vi "Find Entity by ID.vi"(7 "Entity Type":refnum<class "Entity.lvclass">, 8 "error in (no error)":errorcluster, 10 "Entity ID":T1, 11 "Entity Manager in":refnum<class "Entity Manager.lvclass">) -> (0 "error out":errorcluster, 2 "Entity":refnum<class "Entity.lvclass">, 3 "Entity Manager out":refnum<class "Entity Manager.lvclass">)   [LabVIEW 2020, in "Conditu2.lvlib" / "Entity Manager.lvclass"]
uses:
  Entity Manager.lvclass
  Entity/Entity.lvclass
  Entity ID.ctl
  Entity Manager.lvclass/Entity Manager.ctl
  Unit Of Work Session/Unit Of Work Session.lvclass
  Conditu2.lvlib
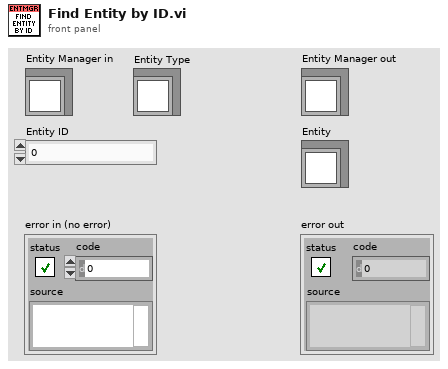
[diagram p1: front panel]
types:
  T1 = typedef "Conditu2.lvlib/Entity ID.ctl" = i64
  T2 = typedef "Conditu2.lvlib/Entity Manager.lvclass/Entity Info.ctl" = cluster{"Entity":refnum<class "Entity.lvclass">, "Types":refnum<class "Type.lvclass">[], "Type Name Map":map{string, i32}, "Has Relation":bool}
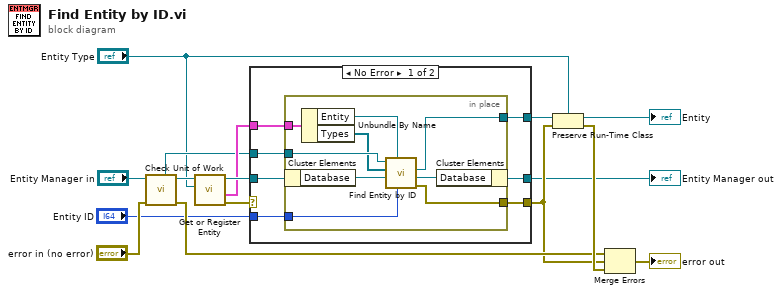
[diagram p0: block diagram]
diagram:
  n1 = call "Check Unit of Work.vi"("error in (no error)"="error in (no error)", "Entity Manager in"="Entity Manager in") -> ("error out"=w15:errorcluster, "Entity Manager out"=w4:refnum<class "Entity Manager.lvclass">, "Unit Of Work"=w3:refnum<class "Unit Of Work Session.lvclass">)  [unwired: 7 in]
  n2 = call "Get or Register Entity.vi"("Entity"="Entity Type", "Entity Manager in"=w4) -> ("error out"=w7:errorcluster, "Entity Info"=w9:T2, "Entity Manager out"=w10:refnum<class "Entity Manager.lvclass">)  [unwired: 7 in]
  n3 = case shown="No Error" w7 {
    selector: w7 -> [_ w34]
    tunnel: [w17 w34] -> w13
    tunnel: "Entity ID" -> [w23 _]
    tunnel: [w22 w33] -> w11
    tunnel: w10 -> [w20 w33]
    tunnel: w9 -> [w21 _]
    tunnel: w3 -> [w19 _]
    tunnel: [w18 _] -> w1
    frame No Error {
      n4 = in-place {
        in-place-border: w23 -> [w29]
        in-place-border: w21 -> [w32]
        in-place-border: w19 -> [w30]
        in-place-border: [w27] -> w18
        in-place-border: [w28] -> w17
        n5 = in-place-cluster #1(w20) -> ("Database"=w24:refnum<class "Database Platform.lvclass">)
        n6 = Unbundle By Name(w32) -> ("Entity"=w31:refnum<class "Entity.lvclass">, "Types"=w25:refnum<class "Type.lvclass">[])
        n7 = call "Find Entity by ID.vi"("Entity ID"=w29, "Entity Type"=w31, "Database in"=w24, "Types"=w25, "Unit Of Work in"=w30) -> ("error out"=w28:errorcluster, "Database out"=w26:refnum<class "Database Platform.lvclass">, "Entity"=w27:refnum<class "Entity.lvclass">)  [unwired: 4 in]
        n8 = in-place-cluster #1("Database"=w26) -> (w22:refnum<class "Entity Manager.lvclass">)
      }
    }
    frame Error {
    }
  }
  "Entity Manager out" <- w11
  n9 = Preserve Run-Time Class(object in=w1, error in=w13, 2:"Entity Type") -> (object out=→"Entity":refnum<class "Entity.lvclass">, error out=w16:errorcluster)
  n10 = Merge Errors(w15, w13, w16) -> (→"error out":errorcluster)
